vi "FixupVimLinkage.vi"   [LabVIEW 2020]
uses:
  <vilib>/Utility/traverseref.llb/TRef TravTarget.ctl
  4f3c976a-d1c1-4c22-941c-dd3f992a0953.vi
  <vilib>/Utility/traverseref.llb/VI Scripting - Traverse.lvlib
types:
  T1 = typedef "TRef TravTarget.ctl" = enum16{"FP", "BD", "Other"}
  T2 = enum32{"Invalid", "Standard", "Closed", "Hidden", "Minimized", "Maximized"}
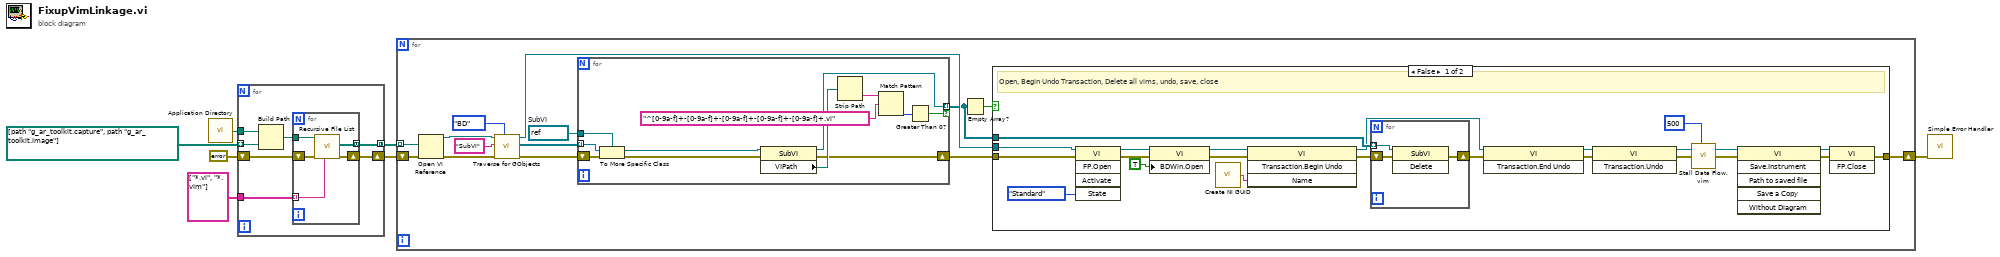
[diagram p0: block diagram]
diagram:
  n1 = call <vilib>:"Application Directory.vi"() -> ("Application Directory"=w1:path)
  n2 = for {
    tunnel: string[] ["*.vi", "*.vim"] ("pattern") -> [w14]
    tunnel: [w13] -> w6 mode=concatenating
    shift-right: [w12] -> w3
    shift-left: errorcluster {"status"=FALSE, "code"=0, "source"=""} ("error constant") -> [w11]
    tunnel: path[] [path "g_ar_toolkit.capture", path "g_ar_toolkit.image"] ("name or relative path") -> [w10] mode=indexing
    tunnel: w1 -> [w9]
    n3 = Build Path(base path=w9, name or relative path=w10) -> (appended path=w8:path)
    n4 = for {
      tunnel: w14 -> [w19] mode=indexing
      tunnel: [w18] -> w13 mode=concatenating
      tunnel: w8 -> [w15]
      shift-right: [w17] -> w12
      shift-left: w11 -> [w16]
      n5 = call <vilib>:"Recursive File List.vi"("pattern"=w19, "error in (no error)"=w16, "Folder Path"=w15) -> ("error out"=w17:errorcluster, "All Files in Dir"=w18:path[])  [unwired: 4 in, 3 out]
    }
  }
  n6 = for {
    tunnel: w6 -> [w20] mode=indexing
    shift-right: [w22] -> w4
    shift-left: w3 -> [w21]
    w29 = refnum<vi> refnum  # SubVI
    n7 = Open VI Reference(vi path=w20, error in (no error)=w21) -> (vi reference=w23:refnum<vi>, error out=w24:errorcluster)  [unwired: 4 in]
    n8 = call <vilib>:"Traverse for GObjects.vi"("Traverse Target"=TRef_TravTarget."BD", "error in (no error)"=w24, "Class Name"="SubVI", "VI Refnum"=w23) -> ("error out"=w30:errorcluster, "References"=w32:refnum<vi>[], "dup VI Refnum"=w26:refnum<vi>)  [unwired: 4 in, 1 out]
    n9 = for {
      tunnel: w32 -> [w70] mode=indexing
      shift-right: [w60] -> w27
      shift-left: w30 -> [w71]
      tunnel: w29 -> [w69]
      tunnel: [w66] -> w25 mode=indexing if=w61
      n10 = To More Specific Class(target class=w69, reference=w70, error in=w71) -> (specific class reference=w67:refnum<vi>, error out=w68:errorcluster)
      n11 = property class="SubVI"(reference=w67, error in=w68) -> (reference out=w66:refnum<vi>, error out=w60:errorcluster, "VIPath"=w65:path)
      n12 = Strip Path(path=w65) -> (name=w64:string)  [unwired: 1 out]
      n13 = Match Pattern(string=w64, regular expression="^[0-9a-f]+-[0-9a-f]+-[0-9a-f]+-[0-9a-f]+-[0-9a-f]+.vi") -> (offset past match=w62:i32)  [unwired: 1 in, 3 out]
      n14 = Greater Than 0?(x=w62) -> (x > 0?=w61:bool)
    }
    n15 = Empty Array?(array=w25) -> (empty?=w28:bool)
    n16 = case shown="False" w28 {
      tunnel: w27 -> [w44 w59]
      tunnel: w26 -> [w45 _]
      tunnel: w25 -> [w54 _]
      tunnel: [w40 w59] -> w22
      frame False {
        # "Open, Begin Undo Transaction, Delete all vims, undo, save, close"
        n17 = invoke class="VI" method="FP.Open"(reference=w45, error in=w44, "State"=T2."Standard") -> (reference out=w39:refnum<vi>, error out=w43:errorcluster)  [unwired: 2 in, 3 out]
        n18 = property class="VI"(reference=w39, error in=w43, "BDWin.Open"=TRUE ("Block Diagram Window:Open")) -> (reference out=w38:refnum<vi>, error out=w34:errorcluster)
        n19 = call <vilib>:"Create NI GUID.vi"() -> ("NI GUID"=w55:string)
        n20 = invoke class="VI" method="Transaction.Begin Undo"(reference=w38, error in=w34, "Name"=w55) -> (reference out=w51:refnum<vi>, error out=w53:errorcluster)  [unwired: 1 in, 2 out]
        n21 = for {
          tunnel: w54 -> [w58] mode=indexing
          shift-right: [w56] -> w52
          shift-left: w53 -> [w57]
          n22 = invoke class="SubVI" method="Delete"(reference=w58, error in=w57) -> (error out=w56:errorcluster)  [unwired: 1 in, 2 out]
        }
        n23 = invoke class="VI" method="Transaction.End Undo"(reference=w51, error in=w52) -> (reference out=w50:refnum<vi>, error out=w49:errorcluster)  [unwired: 1 in, 1 out]
        n24 = invoke class="VI" method="Transaction.Undo"(reference=w50, error in=w49) -> (reference out=w48:refnum<vi>, error out=w47:errorcluster)  [unwired: 1 in, 1 out]
        n25 = call "Stall Data Flow.vim"("value in"=w47, "milliseconds to wait"=u32 500) -> ("value out"=w36:errorcluster)  [unwired: 1 out]
        n26 = invoke class="VI" method="Save.Instrument"(reference=w48, error in=w36) -> (reference out=w42:refnum<vi>, error out=w41:errorcluster)  [unwired: 4 in, 4 out]
        n27 = invoke class="VI" method="FP.Close"(reference=w42, error in=w41) -> (error out=w40:errorcluster)  [unwired: 1 in, 2 out]
      }
      frame True {
        # "no vims"
      }
    }
  }
  n28 = call <vilib>:"Simple Error Handler.vi"("error in (no error)"=w4) -> ()  [unwired: 4 in, 5 out]
